vi "Init (Raw).vi"(6 "Index (:TODO:)":i32=-1, 8 "error in (no error)":errorcluster, 10 "Data":string[](array[string])) -> (0 "error out":errorcluster, 3 "Find First Query out":refnum<class "Insert Query.lvclass">)   [LabVIEW 2013, in "Insert Query.lvclass"]
doc: "Copyright 2018, Carya Automatisering, Wiebe Walstra."
uses:
  Insert Query.lvclass
  Insert Query.lvclass/Insert Query.ctl
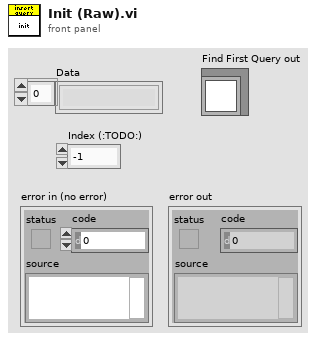
[diagram p1: front panel]
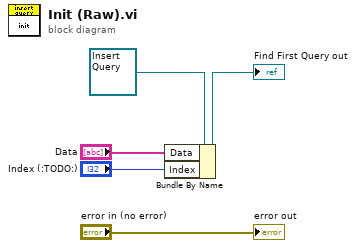
[diagram p0: block diagram]
diagram:
  n1 = Bundle By Name(cluster=refnum<class "Insert Query.lvclass"> refnum ("Find First Query in"), "Data"="Data", "Index"="Index (:TODO:)") -> (→"Find First Query out":refnum<class "Insert Query.lvclass">)
  "error out" <- "error in (no error)"
